vi "Collections.vi"(8 "error in (no error)":errorcluster, 11 "Node Ptr":T1 format="%.0x") -> (0 "error out":errorcluster)   [LabVIEW 2024, in "Diagnostics Addon System Explorer.lvlib"]
uses:
  Diagnostics Addon System Explorer.lvlib
  <vilib>/NI VeriStand/Custom Device API/Custom Device Item Ref.ctl
  Types/FG.Action.ctl
  Addon Shared/SubVIs/Constants.vi
  <vilib>/NI/NI VeriStand Advanced SysDef API/SysDef API/SysDef.Property.Set.vi
  <vilib>/NI/NI VeriStand Advanced SysDef API/_SubVIs/SysDef.Property.Set.U32.vi
  <vilib>/NI VeriStand/Custom Device API/NI VeriStand - Get Item Property.vi
  <vilib>/NI VeriStand/Custom Device API/Get Item Property (U32).vi
  <vilib>/NI VeriStand/Custom Device API/Custom Device API.lvlib
  Addon Shared/Diagnostics Addon Shared.lvlib
panel:
  in  "SHDocVw.IWebBrowser":refnum<k7>(container)
  in  "Collection":i32(listbox) caption="Collections"
  in  "Description":string
  out "Name":string
  in  "Header":cluster{"Section Name":string}={"Section Name"="Collection Settings"}
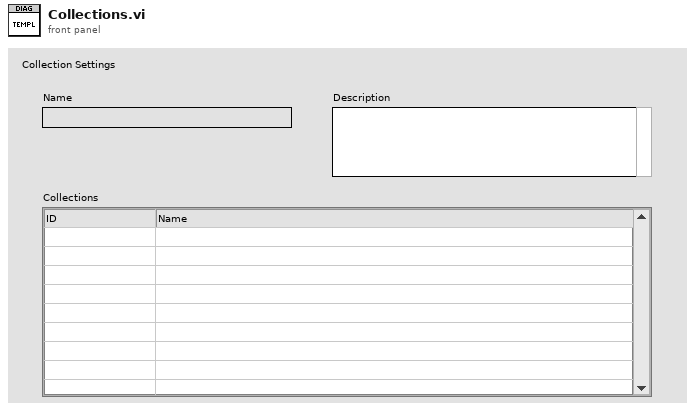
[diagram p1: front panel]
types:
  T1 = typedef "Custom Device API.lvlib/Custom Device Item Ref.ctl" = u64
  T2 = typedef "Diagnostics Addon System Explorer.lvlib/FG.Action.ctl" = enum16{"Get", "Set"}
  T3 = typedef "Custom Device API.lvlib/Custom Device Item Info.ctl" = cluster{"Name":string, "Is Channel":bool, "GUID":string, "Is Waveform":bool}
  T4 = typedef "Custom Device API.lvlib/Custom Device Commands.ctl" = enum16{"Default", "Item renamed", "Shutdown", "Dynamic button pressed"}
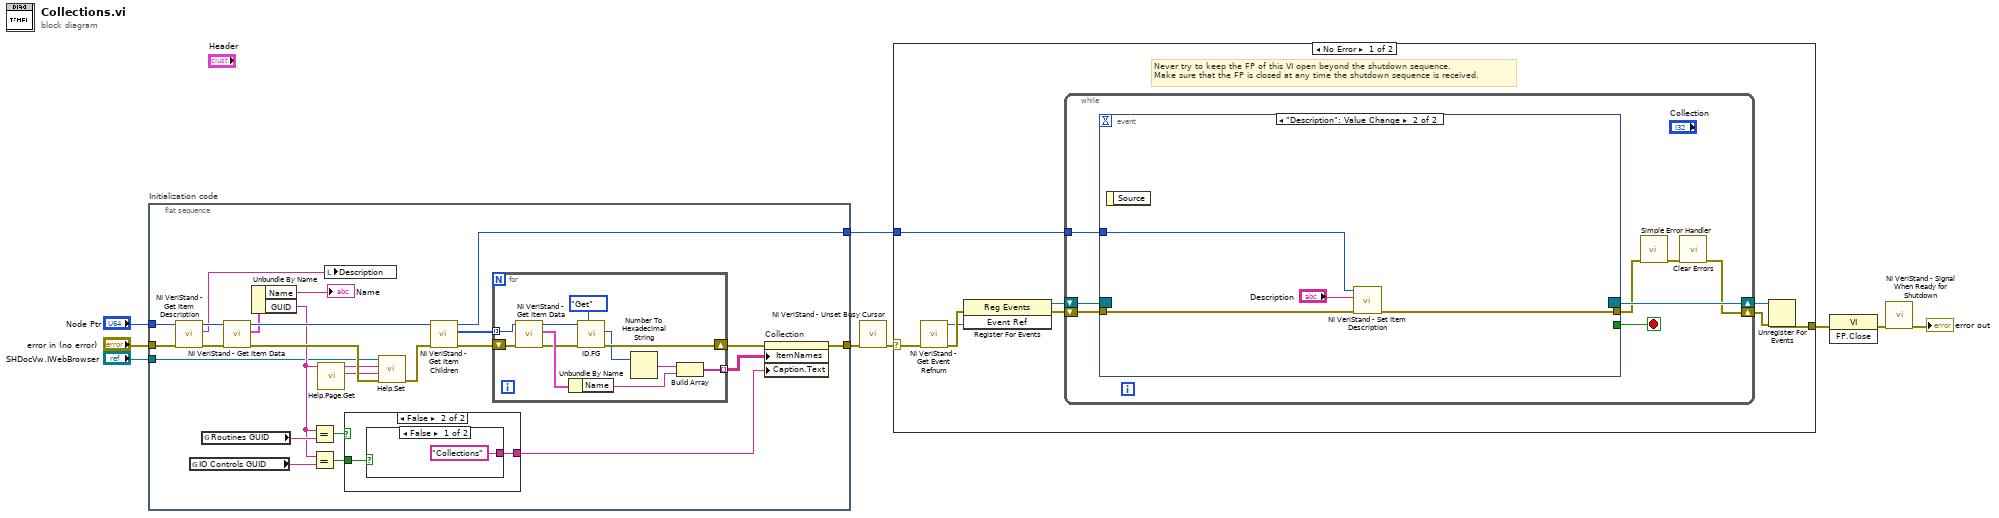
[diagram p0: block diagram]
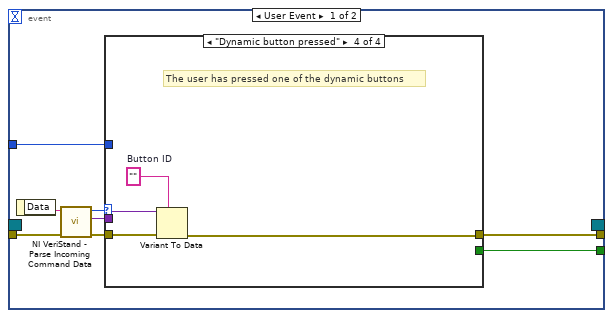
[diagram p2: hidden frame]
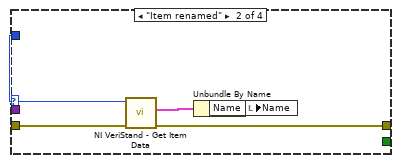
[diagram p4: hidden frame]
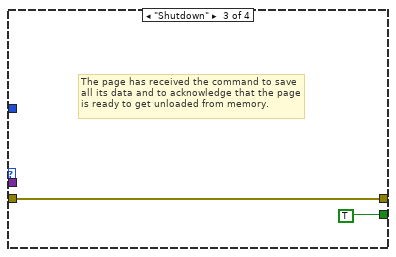
[diagram p5: hidden frame]
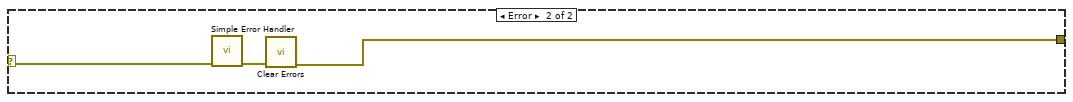
[diagram p6: hidden frame]
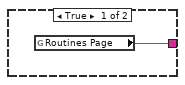
[diagram p7: hidden frame]
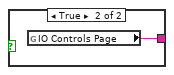
[diagram p8: hidden frame]
diagram:
  n1 = flat-sequence "Initialization code" {
    tunnel: "error in (no error)" -> [w11]
    tunnel: [w24] -> w6
    tunnel: [w26] -> w3
    tunnel: "Node Ptr" -> [w29]
    tunnel: "SHDocVw.IWebBrowser" -> [w12]
    frame #0 {
      n2 = call <vilib>:"NI VeriStand - Get Item Description.vi"("error in (no error)"=w11, "Item Ref in"=w29) -> ("error out"=w31:errorcluster, "Description"=w32:string, "Item Ref out"=w33:T1)  [unwired: 7 out]
      n3 = global read "Constants.vi" "IO Controls GUID"() -> (w20:string)
      n4 = global read "Constants.vi" "Routines GUID"() -> (w21:string)
      n5 = call <vilib>:"NI VeriStand - Get Item Data.vi"("error in (no error)"=w31, "Item Ref in"=w33) -> ("error out"=w16:errorcluster, "Item Info"=w30:T3, "Item Ref out"=w34:T1)  [unwired: 7 out]
      n6 = Unbundle By Name(w30) -> ("Name"=→"Name":string, "GUID"=w13:string)
      n7 = Equal?(x=w13, y=w21) -> (x = y?=w19:bool)
      n8 = Equal?(x=w13, y=w20) -> (x = y?=w17:bool)
      n9 = call "Help.Page.Get.vi"("GUID"=w13) -> ("HTML File"=w14:string, "Main CHM File"=w10:string)  [unwired: 9 in]
      n10 = local write "Description"(w32) -> ()
      n11 = case shown="False" w19 {
        tunnel: [w35 w37] -> w18
        tunnel: w17 -> [_ w36]
        frame True {
          n12 = global read "Constants.vi" "Routines Page"() -> (w35:string)
        }
        frame False {
          n13 = case shown="False" w36 {
            tunnel: ["Collections" ("IO Controls Page") w39] -> w37
            frame False {
            }
            frame True {
              n14 = global read "Constants.vi" "IO Controls Page"() -> (w39:string)
            }
          }
        }
      }
      n15 = call "Help.Set.vi"("error in (no error)"=w16, "HTML File"=w14, "Main CHM File"=w10, "SHDocVw.IWebBrowser2"=w12) -> ("error out"=w15:errorcluster)  [unwired: 7 in]
      n16 = call <vilib>:"NI VeriStand - Get Item Children.vi"("error in (no error)"=w15, "Item Ref in"=w34) -> ("error out"=w28:errorcluster, "Child Refs"=w27:T1[], "Item Ref out"=w26:T1)  [unwired: 6 in, 1 out]
      n17 = for {
        shift-right: [w43] -> w25
        shift-left: w28 -> [w50]
        tunnel: w27 -> [w49] mode=indexing
        tunnel: [w46] -> w23 mode=indexing
        n18 = call <vilib>:"NI VeriStand - Get Item Data.vi"("error in (no error)"=w50, "Item Ref in"=w49) -> ("error out"=w44:errorcluster, "Item Info"=w48:T3, "Item Ref out"=w42:T1)  [unwired: 7 out]
        n19 = Unbundle By Name(w48) -> ("Name"=w47:string)
        n20 = call "ID.FG.vi"("Action"=FG.Action."Get", "error in (no error)"=w44, "Device Item Ref in"=w42) -> ("error out"=w43:errorcluster, "ID"=w41:u32)  [unwired: 6 in, 1 out]
        n21 = Number To Hexadecimal String(2:w41) -> (0:w45:string)  [unwired: 1 in]
        n22 = Build Array(w45, w47) -> (w46:string[])
      }
      n23 = property on="Collection" class="MCListbox (strict)"(error in=w25, "ItemNames"=w23, "Caption.Text"=w18) -> (error out=w24:errorcluster)  [unwired: 1 in, 1 out]
    }
  }
  n24 = call <vilib>:"NI VeriStand - Unset Busy Cursor.vi"("error in (no error)"=w6) -> ("error out"=w5:errorcluster)  [unwired: 10 out]
  n25 = case shown="No Error" w5 {
    selector: w5 -> [w51 w94]
    tunnel: [w56 w92] -> w9
    tunnel: w3 -> [w52 _]
    frame No Error {
      # "Never try to keep the FP of this VI open beyond the shutdown sequence.\nMake sure that the FP is closed at any time the shutdown sequence is received."
      n26 = call <vilib>:"NI VeriStand - Get Event Refnum.vi"("error in (no error)"=w51) -> ("error out"=w59:errorcluster, "Event Ref"=w55:refnum<user-event>)  [unwired: 9 out]
      n27 = register-events(error in=w59, w55) -> (reference out=w53:refnum<event-registration>, error out=w54:errorcluster)  [unwired: 1 in]
      n28 = while {
        tunnel: w52 -> [w63]
        shift-right: [w60] -> w57
        shift-left: w54 -> [w66]
        shift-right: [w67] -> w58
        shift-left: w53 -> [w65]
        stop <- w64 stop-if-true
        n29 = event shown="[1] \"Description\": Value Change" {
          selector: w65 -> [_ _]
          dyn-events: [_ _] -> w67
          timeout: _ -> [_ _]
          tunnel: w66 -> [w75 w90]
          tunnel: [w71 _] -> w64
          tunnel: [w70 w89] -> w62
          tunnel: w63 -> [w69 w91]
          event User Event {
            n30 = event-data() -> ("Data"=w74:string)  [unwired: 1 out]
            n31 = call <vilib>:"NI VeriStand - Parse Incoming Command Data.vi"("error in (no error)"=w75, "Incoming data"=w74) -> ("error out"=w73:errorcluster, "Outgoing data"=w68:variant, "Action"=w72:T4)  [unwired: 7 out]
            n32 = case shown="\"Dynamic button pressed\"" w72 {
              tunnel: w73 -> [w76 w81 w82 w87]
              tunnel: [_ _ TRUE _] -> w71
              tunnel: [w76 w78 w82 w84] -> w70
              tunnel: w69 -> [_ w80 _ _]
              tunnel: w68 -> [_ _ _ w86]
              frame "Default", Default {
              }
              frame "Item renamed" {
                n33 = call <vilib>:"NI VeriStand - Get Item Data.vi"("error in (no error)"=w81, "Item Ref in"=w80) -> ("error out"=w78:errorcluster, "Item Info"=w79:T3)  [unwired: 8 out]
                n34 = Unbundle By Name(w79) -> ("Name"=w77:string)
                n35 = local write "Name"(w77) -> ()
              }
              frame "Shutdown" {
                # "The page has received the command to save all its data and to acknowledge that the page is ready to get unloaded from memory."
              }
              frame "Dynamic button pressed" {
                w85 = ""  # Button ID
                # "The user has pressed one of the dynamic buttons"
                n36 = Variant To Data(error in=w87, type=w85, Variant=w86) -> (error out=w84:errorcluster)  [unwired: 1 out]
              }
            }
          }
          event "Description": Value Change {
            n37 = event-data() -> ()  [unwired: 2 out]
            n38 = call <vilib>:"NI VeriStand - Set Item Description.vi"("error in (no error)"=w90, "Description"="Description", "Item Ref in"=w91) -> ("error out"=w89:errorcluster)  [unwired: 8 out]
          }
        }
        n39 = call <vilib>:"Simple Error Handler.vi"("error in (no error)"=w62) -> ("error out"=w61:errorcluster)  [unwired: 1 in, 7 out]
        n40 = call <vilib>:"Clear Errors.vi"("error in (no error)"=w61) -> ("error out"=w60:errorcluster)  [unwired: 1 in, 5 out]
      }
      n41 = Unregister For Events(event registration refnum=w58, error in=w57) -> (error out=w56:errorcluster)
    }
    frame Error {
      n42 = call <vilib>:"Simple Error Handler.vi"("error in (no error)"=w94) -> ("error out"=w93:errorcluster)  [unwired: 1 in, 7 out]
      n43 = call <vilib>:"Clear Errors.vi"("error in (no error)"=w93) -> ("error out"=w92:errorcluster)  [unwired: 1 in, 5 out]
    }
  }
  n44 = invoke class="VI" method="FP.Close"(error in=w9) -> (error out=w8:errorcluster)  [unwired: 2 in, 2 out]
  n45 = call <vilib>:"NI VeriStand - Signal When Ready for Shutdown.vi"("error in (no error)"=w8) -> ("error out"=→"error out":errorcluster)  [unwired: 10 out]
